vi "Capacity.vi"(0 "Conrtols Valves":T1, 1 "Testing":bool, 2 "Cycle":string(combo)="Cycle 1", 5 "Conrtols AUX":T2, 7 "Exit":bool, 9 "NI1":tag, 11 "NI2":tag) -> (4 "Pressure Sensors 2":T3 {"P5" format="%#.2g"; "P4" format="%#.2g"; "P3" format="%#.2g"; "P2" format="%#.2g"; "P1" format="%#.2g"}, 6 "Temperature Sensors":T4 {"T11" format="%#.2g"; "T10" format="%#.2g"; "T9" format="%#.2g"; "T8" format="%#.2g"; "T7" format="%#.2g"; "T6" format="%#.2g"; "T5" format="%#.2g"; "T4" format="%#.2g"; "T3" format="%#.2g"; "T2" format="%#.2g"; "T1" format="%#.2g"})   [LabVIEW 2017]
panel:
  out "Compressor T > 80":bool
  out "Compressor P > 20":bool
  in  "Tab Control":enum32{"User Interface"}(tab)
  # "CAPACITY CONTROL AND FAULTS IN REFREGERATION SYSTEM"
  # "Bar"
  # "Bar"
  # "Bar"
  # "Bar"
  # "Bar"
  # "C"
  # "C"
  # "C"
  # "C"
  # "C"
  # "C"
  # "C"
  # "C"
  # "C"
  # "C"
  # "C"
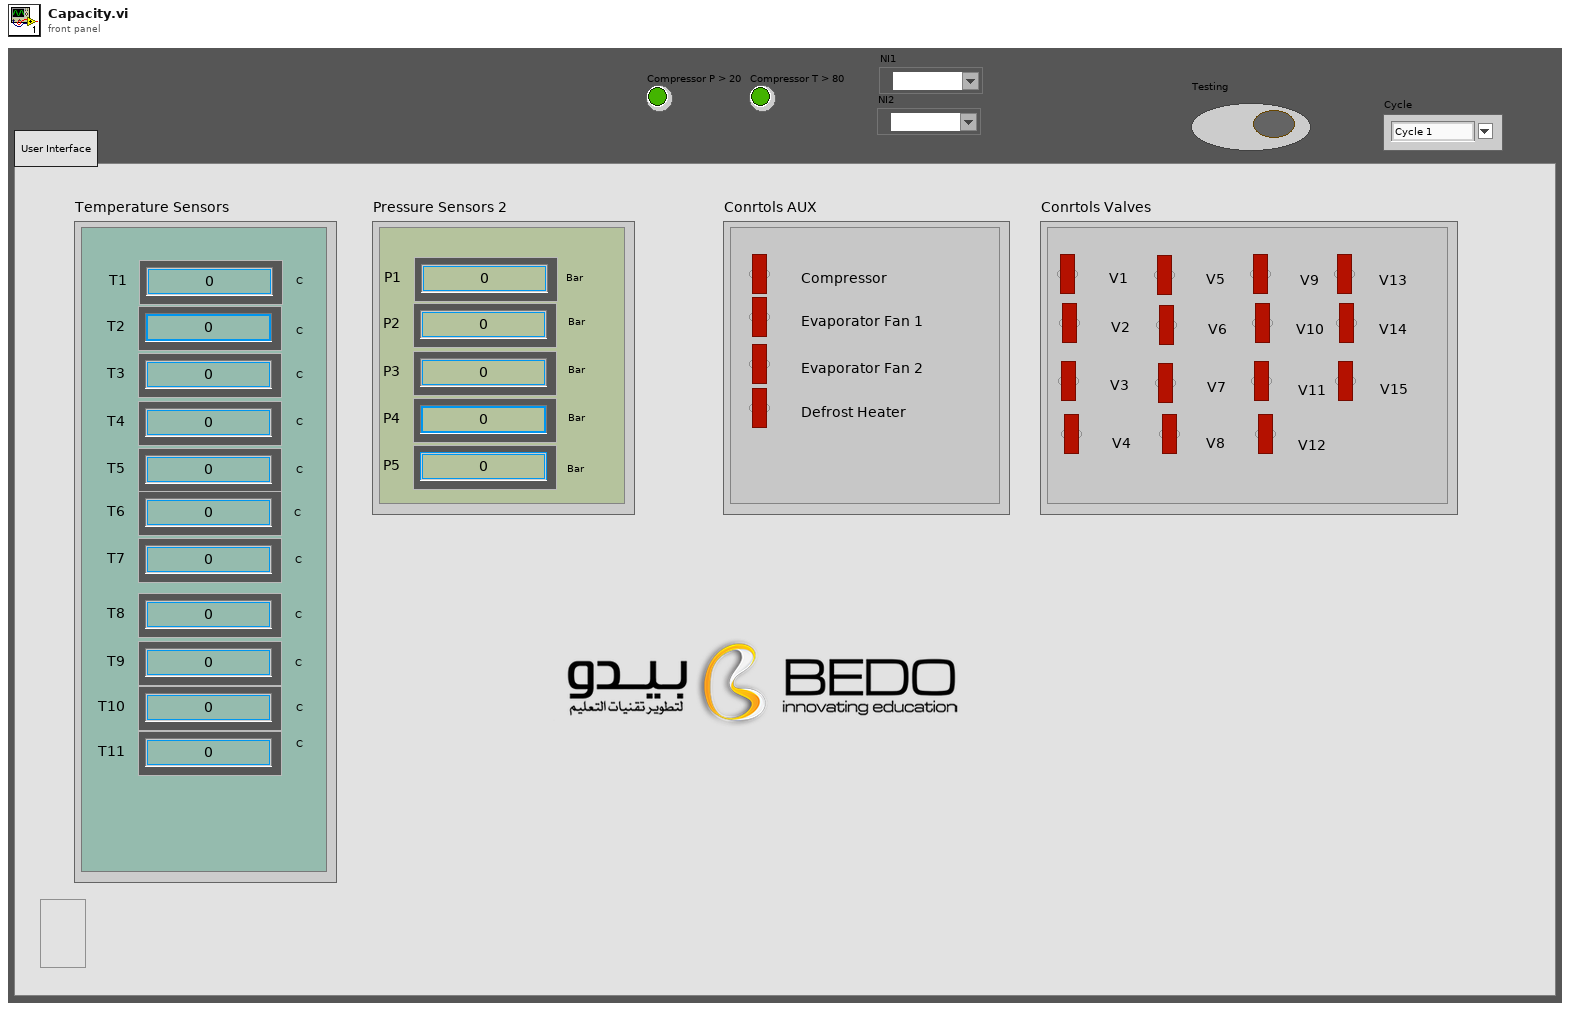
[diagram p1: front panel]
types:
  T1 = cluster{"V1":bool, "V2":bool, "V3":bool, "V4":bool, "V5":bool, "V6":bool, "V7":bool, "V8":bool, "V9":bool, "V10":bool, "V11":bool, "V12":bool, "V13":bool, "V14":bool, "V15":bool}
  T2 = cluster{"Compressor":bool, "Evaporator Fan 1":bool, "Evaporator Fan 2":bool, "Defrost Heater":bool}
  T3 = cluster{"P1":dbl, "P2":dbl, "P3":dbl, "P4":dbl, "P5":dbl}
  T4 = cluster{"T1":dbl, "T2":dbl, "T3":dbl, "T4":dbl, "T5":dbl, "T6":dbl, "T7":dbl, "T8":dbl, "T9":dbl, "T10":dbl, "T11":dbl}
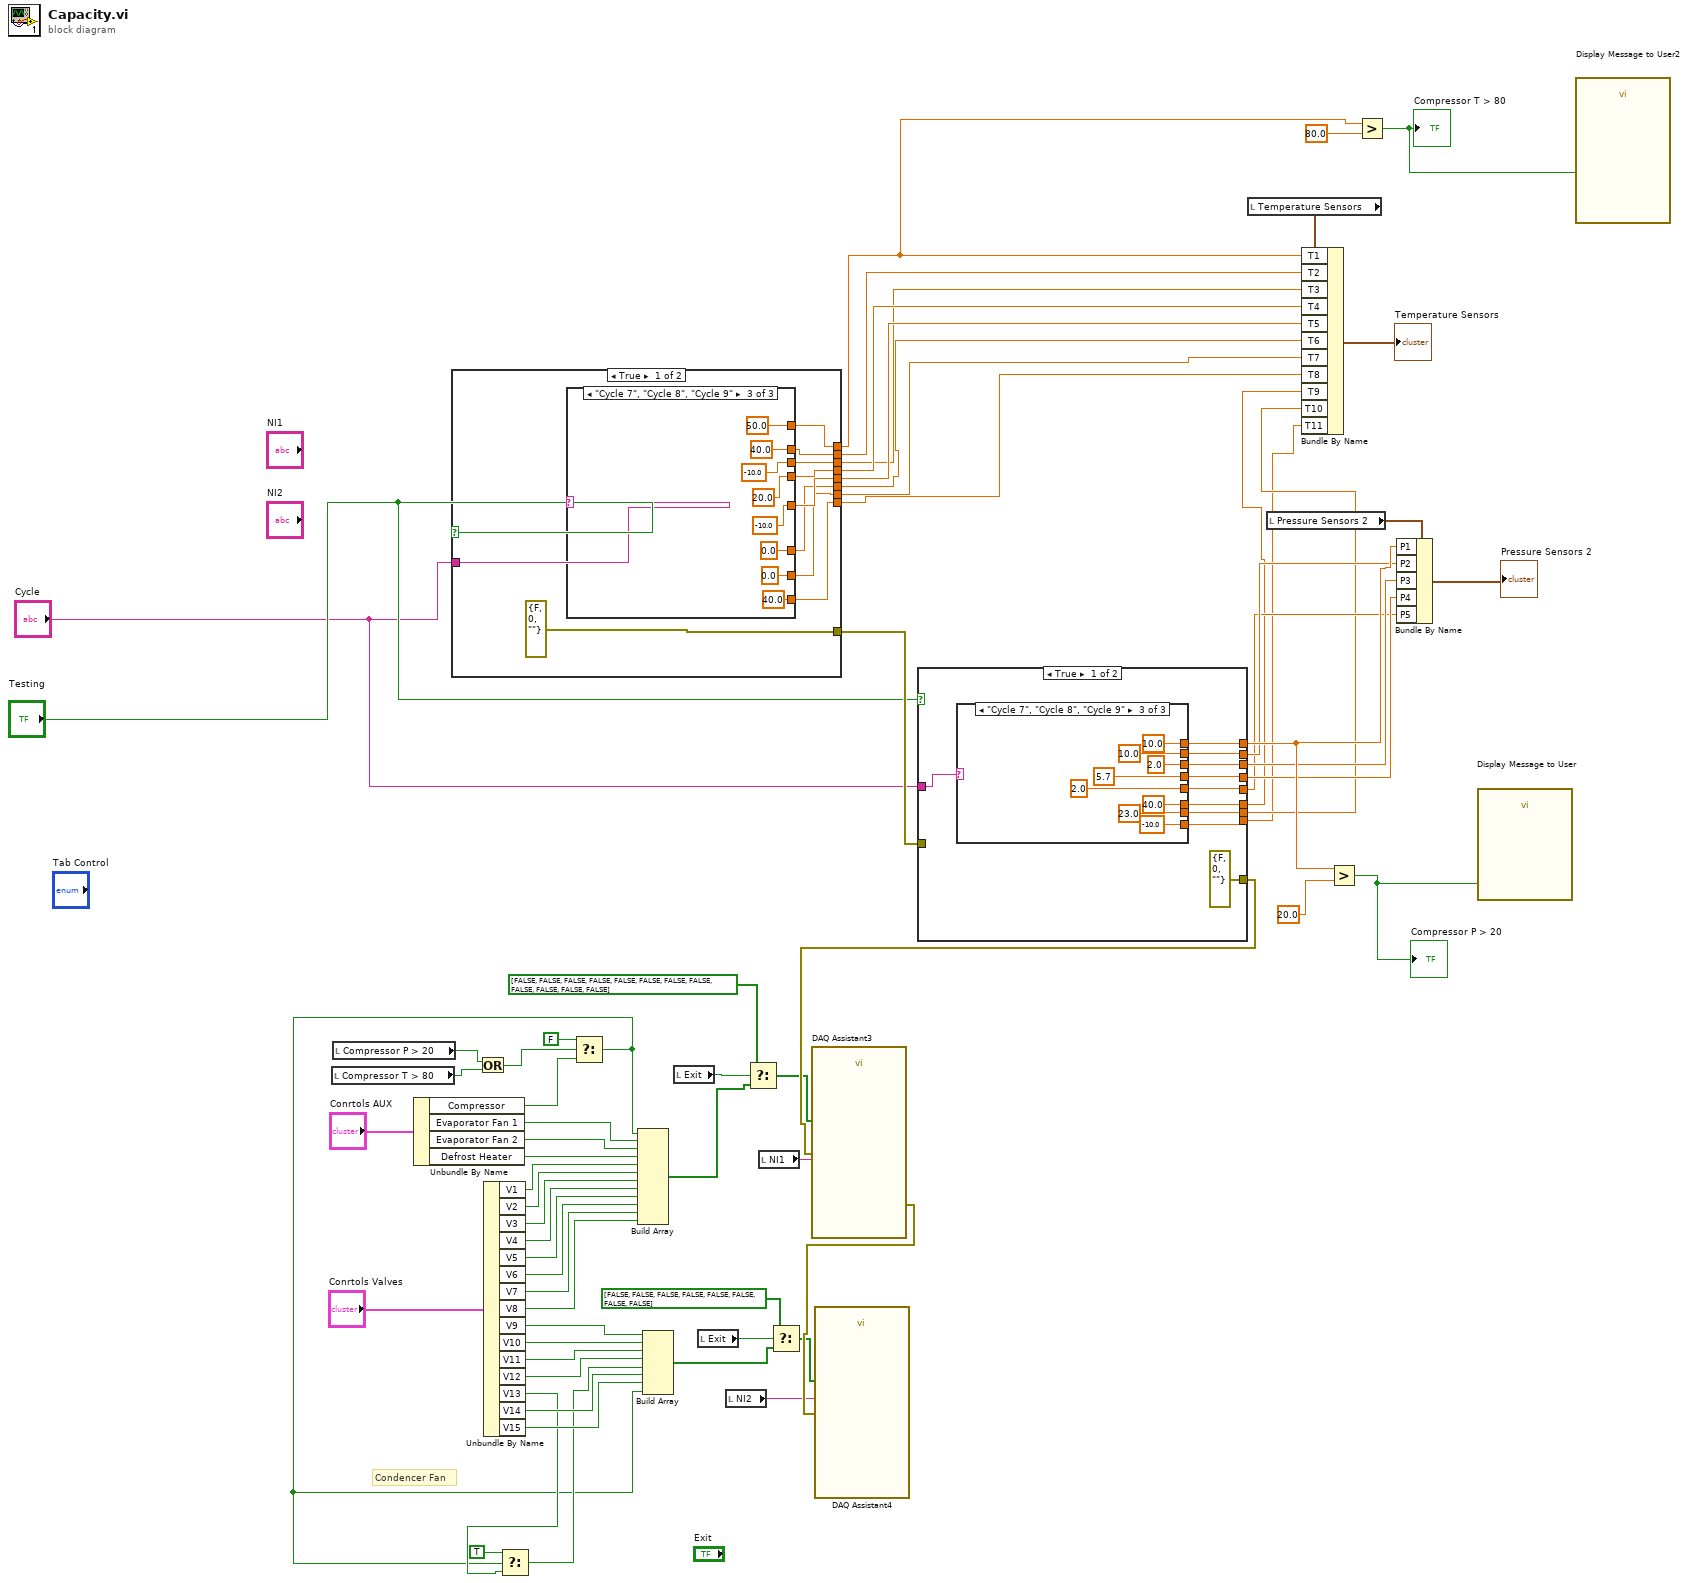
[diagram p0: block diagram]
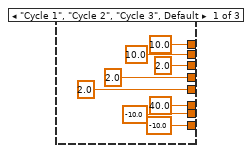
[diagram p2: hidden frame]
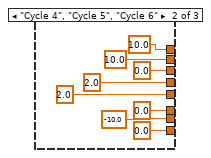
[diagram p3: hidden frame]
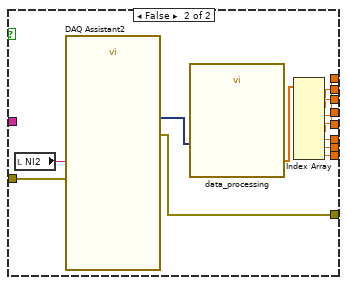
[diagram p4: hidden frame]
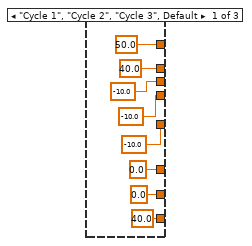
[diagram p5: hidden frame]
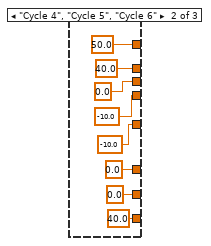
[diagram p6: hidden frame]
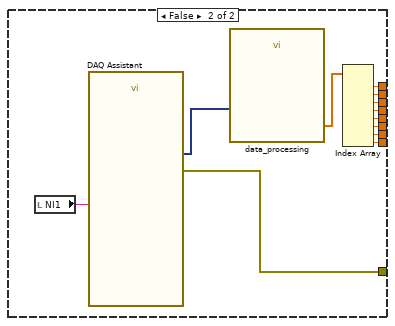
[diagram p7: hidden frame]
diagram:
  # "Condencer Fan"
  n1 = local read "Compressor T > 80"() -> (w21:bool)
  n2 = local read "Compressor P > 20"() -> (w20:bool)
  n3 = Unbundle By Name("Conrtols AUX") -> ("Compressor"=w27:bool, "Evaporator Fan 1"=w47:bool, "Evaporator Fan 2"=w48:bool, "Defrost Heater"=w49:bool)
  n4 = case shown="True" "Testing" {
    tunnel: [errorcluster {"status"=FALSE, "code"=0, "source"=""} ("error out") w112] -> w42
    tunnel: [w77 w109] -> w17
    tunnel: [w76 w108] -> w16
    tunnel: [w75 w107] -> w1
    tunnel: [w74 w106] -> w15
    tunnel: [w73 w105] -> w14
    tunnel: [w72 w104] -> w13
    tunnel: [w71 w103] -> w12
    tunnel: [w70 w102] -> w11
    tunnel: "Cycle" -> [w68 _]
    frame True {
      n5 = case shown="\"Cycle 7\", \"Cycle 8\", \"Cycle 9\"" w68 {
        tunnel: [50.0 ("Scalar") 50.0 ("Scalar") 50.0 ("Scalar")] -> w77
        tunnel: [40.0 ("Scalar") 40.0 ("Scalar") 40.0 ("Scalar")] -> w76
        tunnel: [-10.0 ("Scalar") 0.0 ("Scalar") -10.0 ("Scalar")] -> w75
        tunnel: [-10.0 ("Scalar") -10.0 ("Scalar") 20.0 ("Scalar")] -> w74
        tunnel: [-10.0 ("Scalar") -10.0 ("Scalar") -10.0 ("Scalar")] -> w73
        tunnel: [0.0 ("Scalar") 0.0 ("Scalar") 0.0 ("Scalar")] -> w72
        tunnel: [0.0 ("Scalar") 0.0 ("Scalar") 0.0 ("Scalar")] -> w71
        tunnel: [40.0 ("Scalar") 40.0 ("Scalar") 40.0 ("Scalar")] -> w70
        frame "Cycle 1", "Cycle 2", "Cycle 3", Default {
        }
        frame "Cycle 4", "Cycle 5", "Cycle 6" {
        }
        frame "Cycle 7", "Cycle 8", "Cycle 9" {
        }
      }
    }
    frame False {
      n6 = local read "NI1"() -> (w113:tag)
      n7 = call "DAQ Assistant"("device name"=w113) -> ("data"=w110:dynamicdata, "error out"=w112:errorcluster)  [unwired: 16 in, 1 out]
      n8 = call "data_processing.vi"("data"=w110) -> ("DATA"=w111:dbl[])  [unwired: 10 in]
      n9 = Index Array(array=w111) -> (element #1=w109:dbl, element #2=w108:dbl, element #3=w107:dbl, element #4=w106:dbl, element #5=w105:dbl, element #6=w104:dbl, element #7=w103:dbl, element #8=w102:dbl)  [unwired: 8 in]
    }
  }
  n10 = Or(x=w20, y=w21) -> (x .or. y?=w19:bool)
  n11 = Unbundle By Name("Conrtols Valves") -> ("V1"=w50:bool, "V2"=w51:bool, "V3"=w52:bool, "V4"=w53:bool, "V5"=w54:bool, "V6"=w55:bool, "V7"=w56:bool, "V8"=w57:bool, "V9"=w58:bool, "V10"=w59:bool, "V11"=w60:bool, "V12"=w61:bool, "V13"=w31:bool, "V14"=w62:bool, "V15"=w63:bool)
  n12 = Select(t=FALSE, s=w19, f=w27) -> (s? t:f=w26:bool)
  n13 = Select(t=TRUE, s=w26, f=w31) -> (s? t:f=w30:bool)
  n14 = Build Array(w26, w47, w48, w49, w50, w51, w52, w53, w54, w55, w56, w57) -> (w34:bool[])
  n15 = Build Array(w58, w59, w60, w61, w30, w62, w63, w26) -> (w38:bool[])
  n16 = local read "Exit"() -> (w35:bool)
  n17 = local read "Exit"() -> (w39:bool)
  n18 = local read "NI2"() -> (w45:tag)
  n19 = Select(t=bool[] [FALSE, FALSE, FALSE, FALSE, FALSE, FALSE, FALSE, FALSE, FALSE, FALSE, FALSE, FALSE], s=w35, f=w34) -> (s? t:f=w33:bool[])
  n20 = local read "NI1"() -> (w43:tag)
  n21 = Select(t=bool[] [FALSE, FALSE, FALSE, FALSE, FALSE, FALSE, FALSE, FALSE], s=w39, f=w38) -> (s? t:f=w36:bool[])
  n22 = case shown="True" "Testing" {
    tunnel: [errorcluster {"status"=FALSE, "code"=0, "source"=""} ("error out") w160] -> w66
    tunnel: w42 -> [_ w158]
    tunnel: [w120 w155] -> w10
    tunnel: [w119 w154] -> w9
    tunnel: [w118 w153] -> w8
    tunnel: [w117 w152] -> w7
    tunnel: [w116 w151] -> w6
    tunnel: [w123 w150] -> w5
    tunnel: [w122 w149] -> w4
    tunnel: [w121 w148] -> w3
    tunnel: "Cycle" -> [w114 _]
    frame True {
      n23 = case shown="\"Cycle 7\", \"Cycle 8\", \"Cycle 9\"" w114 {
        tunnel: [40.0 ("Scalar") 0.0 ("Scalar") 40.0 ("Scalar")] -> w123
        tunnel: [-10.0 ("Scalar") -10.0 ("Scalar") 23.0 ("Scalar")] -> w122
        tunnel: [-10.0 ("Scalar") 0.0 ("Scalar") -10.0 ("Scalar")] -> w121
        tunnel: [10.0 ("Scalar") 10.0 ("Scalar") 10.0 ("Scalar")] -> w120
        tunnel: [10.0 ("Scalar") 10.0 ("Scalar") 10.0 ("Scalar")] -> w119
        tunnel: [2.0 ("Scalar") 0.0 ("Scalar") 2.0 ("Scalar")] -> w118
        tunnel: [2.0 ("Scalar") 2.0 ("Scalar") 5.7 ("Scalar")] -> w117
        tunnel: [2.0 ("Scalar") 2.0 ("Scalar") 2.0 ("Scalar")] -> w116
        frame "Cycle 1", "Cycle 2", "Cycle 3", Default {
        }
        frame "Cycle 4", "Cycle 5", "Cycle 6" {
        }
        frame "Cycle 7", "Cycle 8", "Cycle 9" {
        }
      }
    }
    frame False {
      n24 = local read "NI2"() -> (w159:tag)
      n25 = call "DAQ Assistant2"("error in"=w158, "device name"=w159) -> ("data"=w157:dynamicdata, "error out"=w160:errorcluster)  [unwired: 15 in, 1 out]
      n26 = call "data_processing.vi"("data"=w157) -> ("DATA"=w156:dbl[])  [unwired: 10 in]
      n27 = Index Array(array=w156) -> (element #1=w155:dbl, element #2=w154:dbl, element #3=w153:dbl, element #4=w152:dbl, element #5=w151:dbl, element #6=w150:dbl, element #7=w149:dbl, element #8=w148:dbl)  [unwired: 8 in]
    }
  }
  n28 = call "DAQ Assistant3"("data"=w33, "error in"=w66, "device name"=w43) -> ("error out"=w67:errorcluster)  [unwired: 15 in, 1 out]
  n29 = call "DAQ Assistant4"("data"=w36, "error in"=w67, "device name"=w45) -> ()  [unwired: 15 in, 2 out]
  n30 = local read "Temperature Sensors"() -> (w41:T4)
  n31 = local read "Pressure Sensors 2"() -> (w64:T3)
  n32 = Bundle By Name(cluster=w41, "T1"=w17, "T2"=w16, "T3"=w1, "T4"=w15, "T5"=w14, "T6"=w13, "T7"=w12, "T8"=w11, "T9"=w5, "T10"=w4, "T11"=w3) -> (→"Temperature Sensors":T4)
  n33 = Greater?(x=w10, y=20.0) -> (0:w24:bool)
  "Compressor P > 20" <- w24
  n34 = Greater?(x=w17, y=80.0) -> (0:w22:bool)
  "Compressor T > 80" <- w22
  n35 = Bundle By Name(cluster=w64, "P1"=w10, "P2"=w9, "P3"=w8, "P4"=w7, "P5"=w6) -> (→"Pressure Sensors 2":T3)
  n36 = call "Display Message to User"("Enable"=w24) -> ()  [unwired: 9 in, 2 out]
  n37 = call "Display Message to User2"("Enable"=w22) -> ()  [unwired: 9 in, 2 out]
